vi "ni579x Configure EEPROM Write Protection.vi"(0 "Register Bus":T1, 1 "scope":string(combo)="characterization data eeprom", 9 "write protect?":bool, 11 "Error In":errorcluster) -> (4 "Register Bus (out)":T1, 15 "Error Out":errorcluster)   [LabVIEW 2015, in "ni579x Config v2 Host.lvlib"]
uses:
  <instrlib>/ni579x/Config/v2/Host/ni579x Config v2 Host.lvlib
  <instrlib>/_niInstr/Register Bus/v0/Host/Public/Register Bus Session.ctl
  <instrlib>/_niInstr/Register Bus/v0/Host/Private/Session Data.ctl
  <instrlib>/ni579x/Config/v2/Shared/Types/ni579x FAM Register Offset.ctl
  <instrlib>/ni579x/Config/v2/Shared/Types/ni579x FAM Register Operation.ctl
  <instrlib>/ni579x/Config/v2/Shared/ni579x Config v2 Shared.lvlib
  <instrlib>/_niInstr/Register Bus/v0/Host/niInstr Register Bus v0 Host.lvlib
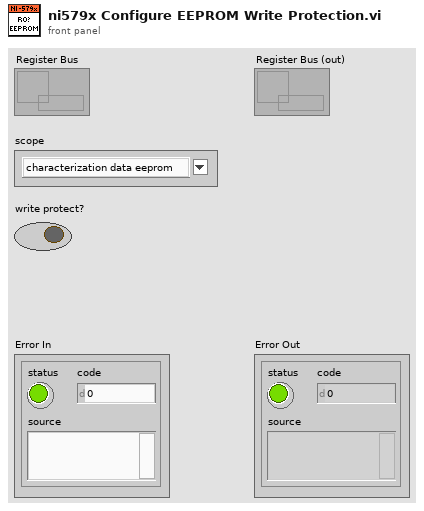
[diagram p1: front panel]
types:
  T1 = typedef "niInstr Register Bus v0 Host.lvlib/Register Bus Session.ctl" = refnum<queue>
  T2 = typedef "ni579x Config v2 Shared.lvlib/ni579x FAM Register Operation.ctl" = cluster{"FAM Register Offset":T3, "Address":u32, "Write (T)/Read (F)":bool, "Write Data":u32}
  T3 = typedef "ni579x Config v2 Shared.lvlib/ni579x FAM Register Offset.ctl" = u8
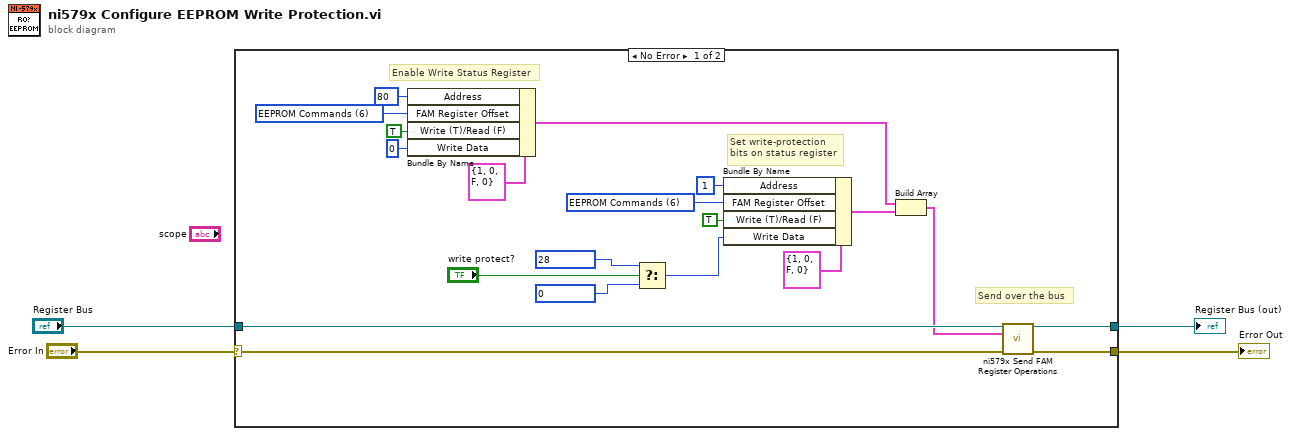
[diagram p0: block diagram]
diagram:
  n1 = case shown="No Error" "Error In" {
    selector: "Error In" -> [w21 w26]
    tunnel: [w23 w26] -> w3
    tunnel: "Register Bus" -> [w22 w25]
    tunnel: [w24 w25] -> w1
    frame No Error {
      w6 = T3 6 items=["ADC"=1, "DAC"=2, "Clock Distribution Chip"=3, "Frequency/Phase Adjust DAC"=4, "EEPROM"=5, "EEPROM Commands"=6, "LO1"=7, "Rx Atten Pre-LNA"=9, "Rx Atten Post-LNA"=10, "Tx Atten"=11] ("FAM Register Offset")
      w7 = T3 6 items=["ADC"=1, "DAC"=2, "Clock Distribution Chip"=3, "Frequency/Phase Adjust DAC"=4, "EEPROM"=5, "EEPROM Commands"=6, "LO1"=7, "Rx Atten Pre-LNA"=9, "Rx Atten Post-LNA"=10, "Tx Atten"=11] ("FAM Register Offset")
      # "Set write-protection\nbits on status register"
      # "Enable Write Status Register"
      # "Send over the bus"
      n2 = Bundle By Name(cluster=T2 {"FAM Register Offset"=1, "Address"=0, "Write (T)/Read (F)"=FALSE, "Write Data"=0} ("FAM Register Operation"), "Address"=u32 80, "FAM Register Offset"=w6, "Write (T)/Read (F)"=TRUE, "Write Data"=u32 0) -> (w11:T2)
      n3 = Select(t=u32 28 ("Write Data"), s="write protect?", f=u32 0 ("Write Data")) -> (s? t:f=w12:u32)
      n4 = Bundle By Name(cluster=T2 {"FAM Register Offset"=1, "Address"=0, "Write (T)/Read (F)"=FALSE, "Write Data"=0} ("FAM Register Operation"), "Address"=u32 1, "FAM Register Offset"=w7, "Write (T)/Read (F)"=TRUE, "Write Data"=w12) -> (w10:T2)
      n5 = Build Array(w11, w10) -> (w9:T2[])
      n6 = call <instrlib>:"ni579x Send FAM Register Operations.vi"("Register Bus"=w22, "FAM Register Operations"=w9, "Error In"=w21) -> ("Register Bus (out)"=w24:T1, "Error Out"=w23:errorcluster)  [unwired: 10 in, 1 out]
    }
    frame Error {
    }
  }
  "Register Bus (out)" <- w1
  "Error Out" <- w3
